vi "ClearStreamId.vi"(8 "error in (no error)":errorcluster, 9 "operating state":string, 10 "data group":string, 11 "OpStateCorrIds in":variant) -> (0 "error out":errorcluster, 2 "operating state corrId":string, 3 "OpStateCorrIds out":variant)   [LabVIEW 2017, in "DataEventCreator.lvlib"]
uses:
  <vilib>/addons/InsightCM/Devices/Shared/Common/DataEventCreator/DataEventCreator.lvlib
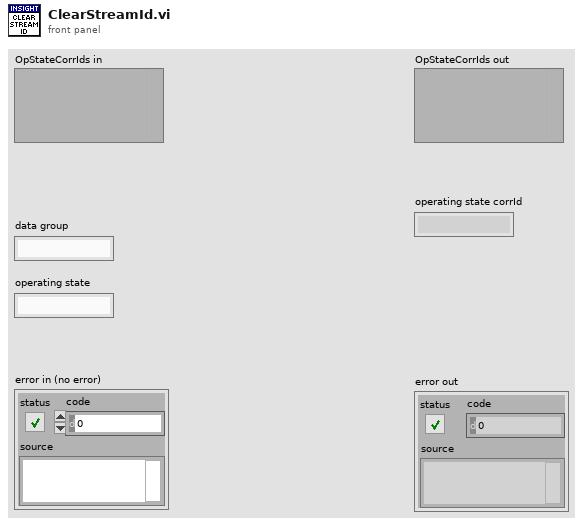
[diagram p1: front panel]
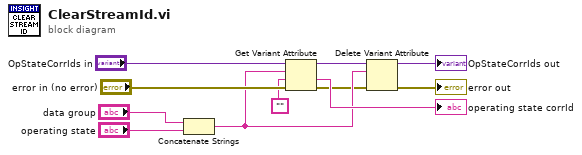
[diagram p0: block diagram]
diagram:
  n1 = Concatenate Strings("data group", "operating state") -> (w3:string)
  n2 = Get Variant Attribute(Variant="OpStateCorrIds in", name=w3, default value (empty Variant)="", error in="error in (no error)") -> (duplicate Variant=w5:variant, value=→"operating state corrId":string, error out=w2:errorcluster)  [unwired: 1 out]
  n3 = Delete Variant Attribute(4:w2, 6:w3, 7:w5) -> (0:→"error out":errorcluster, 3:→"OpStateCorrIds out":variant)  [unwired: 1 out]
